vi "Authenticate without Access Token.vi"(5 "Base URL":string, 6 "Body Parameters":T4[](array[typedef]), 7 "HTTP Method":T5, 8 "error in (no error)":errorcluster, 9 "Header Parameters":T4[](array[typedef]), 10 "URL Parameters":T4[](array[typedef]), 11 "OAuth Handle":T1={"Signature Method"=enum."HMAC-SHA1", "Version"="", "Client"={"Token"="", "Secret"=""}, "Access"={"Token"="", "Secret"=""}}) -> (0 "error out":errorcluster, 1 "Header Value":string, 2 "Header Parameter":string, 3 "Full URL":string, 4 "Body":string)   [LabVIEW 2011, in "i3-oauth.lvlib"]
doc: "Behaves the same as the Authenticate with Access Token VI except that it <b>does not</b> include the Access Credentials as part of the Headers used for the OAuth Signature. <b>This VI SHOULD NOT be used directly in most cases.</b>\n\nThis VI is primarily useful in implementing workflows such as the Browser Workflow Authentication. As of the OAuth 1.0a specification, the only time Access Credentials are unused is when first querying the service using the <b>Request URL</b> and receiving the Temporary Request Credentials to start the process of Authorizing the user."
uses:
  i3-oauth.lvlib
  Controls/Name-Value Pair.ctl
  Controls/HTTP Method.ctl
  Controls/OAuth Handle.ctl
  Controls/Signature Method.ctl
  Controls/Credentials.ctl
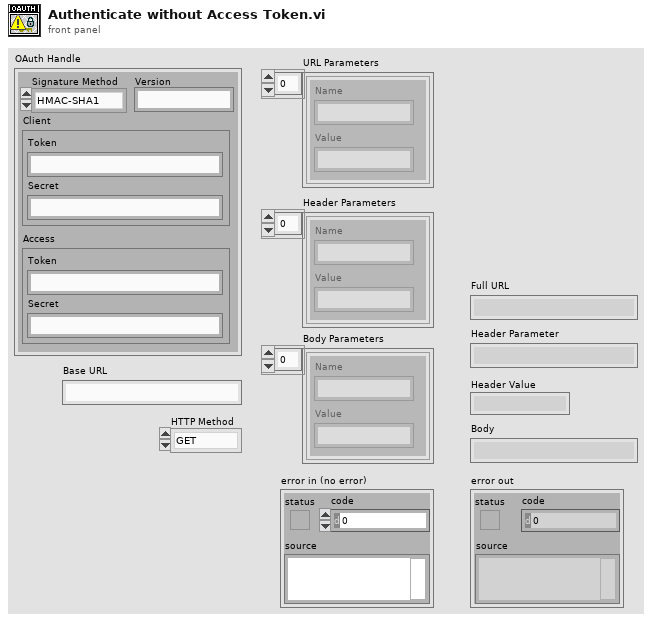
[diagram p1: front panel]
types:
  T1 = typedef "i3-oauth.lvlib/OAuth Handle.ctl" = cluster{"Signature Method":T2, "Version":string, "Client":T3, "Access":T3}
  T2 = typedef "i3-oauth.lvlib/Signature Method.ctl" = enum16{"HMAC-MD5", "HMAC-SHA1", "HMAC-SHA224", "HMAC-SHA256", "HMAC-SHA384", "HMAC-SHA512"}
  T3 = typedef "i3-oauth.lvlib/Credentials.ctl" = cluster{"Token":string, "Secret":string}
  T4 = typedef "i3-oauth.lvlib/Name-Value Pair.ctl" = cluster{"Name":string, "Value":string}
  T5 = typedef "i3-oauth.lvlib/HTTP Method.ctl" = enum16{"GET", "POST", "PUT", "DELETE"}
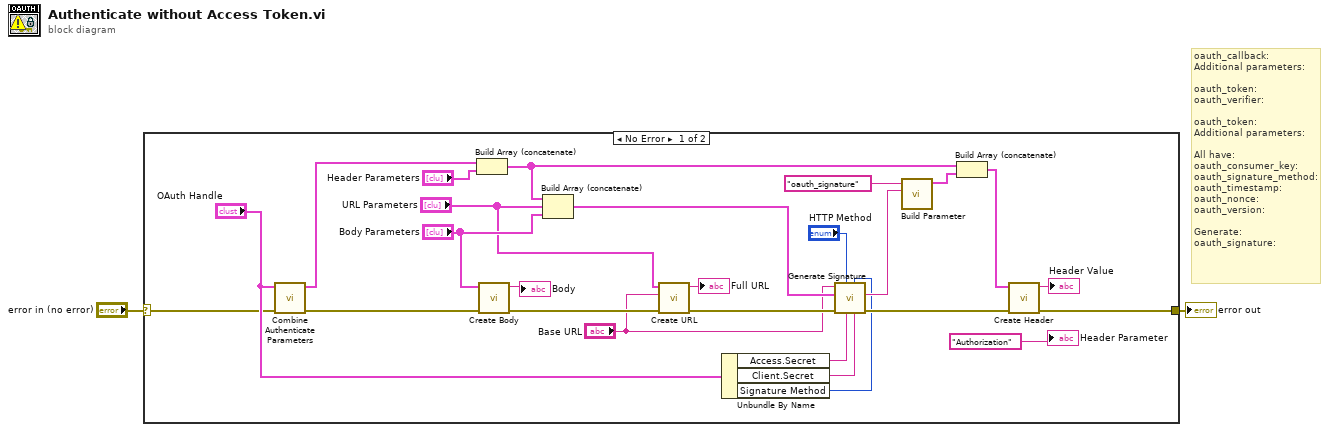
[diagram p0: block diagram]
diagram:
  # "oauth_callback:\nAdditional parameters:\n\noauth_token:\noauth_verifier:\n\noauth_token:\nAdditional parameters:\n\nAll have:\noauth_consumer_key:\noauth_signature_method:\noauth_timestamp:\noauth_nonce:\noauth_version:\n\nGenerate:\noauth_signature:"
  n1 = case shown="No Error" "error in (no error)" {
    selector: "error in (no error)" -> [w5 w29]
    tunnel: [w14 w29] -> w2
    frame No Error {
      n2 = call "Combine Authenticate Parameters.vi"("error in (no error)"=w5, "OAuth Credentials"="OAuth Handle") -> ("error out"=w6:errorcluster, "Authentication Parameters"=w19:T4[])  [unwired: 8 in]
      n3 = Build Array (concatenate)(w19, "Header Parameters") -> (w12:T4[])
      n4 = call "Create Body.vi"("error in (no error)"=w6, "Body Parameters"="Body Parameters") -> ("error out"=w23:errorcluster, "Body"=→"Body":string)  [unwired: 8 in]
      n5 = Build Array (concatenate)(w12, "URL Parameters", "Body Parameters") -> (w27:T4[])
      n6 = call "Create URL.vi"("error in (no error)"=w23, "Base URL"="Base URL", "URL Parameters"="URL Parameters") -> ("error out"=w28:errorcluster, "Full URL"=→"Full URL":string)  [unwired: 7 in]
      n7 = Unbundle By Name("OAuth Handle") -> ("Access.Secret"=w18:string, "Client.Secret"=w17:string, "Signature Method"=w13:T2)
      n8 = call "Generate Signature.vi"("consumer secret"=w17, "Signature Method"=w13, "access token secret"=w18, "HTTP Method"="HTTP Method", "error in (no error)"=w28, "Parameters"=w27, "Base URL"="Base URL") -> ("error out"=w25:errorcluster, "Signature"=w26:string)  [unwired: 3 in]
      n9 = call "Build Parameter.vi"("Value"=w26, "Key"="oauth_signature" ("key")) -> ("Parameter Array"=w9:T4[])  [unwired: 9 in]
      n10 = Build Array (concatenate)(w12, w9) -> (w11:T4[])
      n11 = call "Create Header.vi"("error in (no error)"=w25, "Header Parameters"=w11) -> ("error out"=w14:errorcluster, "Header"=→"Header Value":string)  [unwired: 8 in]
      "Header Parameter" <- "Authorization"
    }
    frame Error {
    }
  }
  "error out" <- w2
